vi "TORC Auto Shift.vi"(6 "RightMotorInput":dbl, 8 "Left Motor Input":dbl format="%#_13g", 9 "Velocity":dbl format="%#_13g", 10 "Throttle":dbl format="%#_13g", 11 "Time Met":bool) -> (3 "Shift Indicator":T1)   [LabVIEW 2015]
uses:
  Shift Enum.ctl
  Team Code/Robot Global Data.vi
  <vilib>/Rock Robotics/WPI/DriverStation/WPI_DriverStationRobotMode2.ctl
panel:
  out "Acceleration Chart":dbl(graph)
  in  "Coast_Speed_Limit":dbl=1.0
  in  "Coast_Throttle_Limit":dbl=0.1
  in  "Dropkik_Speed_Limit":dbl=3.0
  in  "Dropkik_Throttle_limit":dbl=0.3
  in  "Velocity_Upshift_Limit":dbl=3.25
  in  "Accel_up_limit":dbl
  in  "upshift_Thrtl_Limit":dbl=0.5
  in  "ShiftInterval":i32=500
  # "Original Upshift:\n3.75, changed to 3.25"
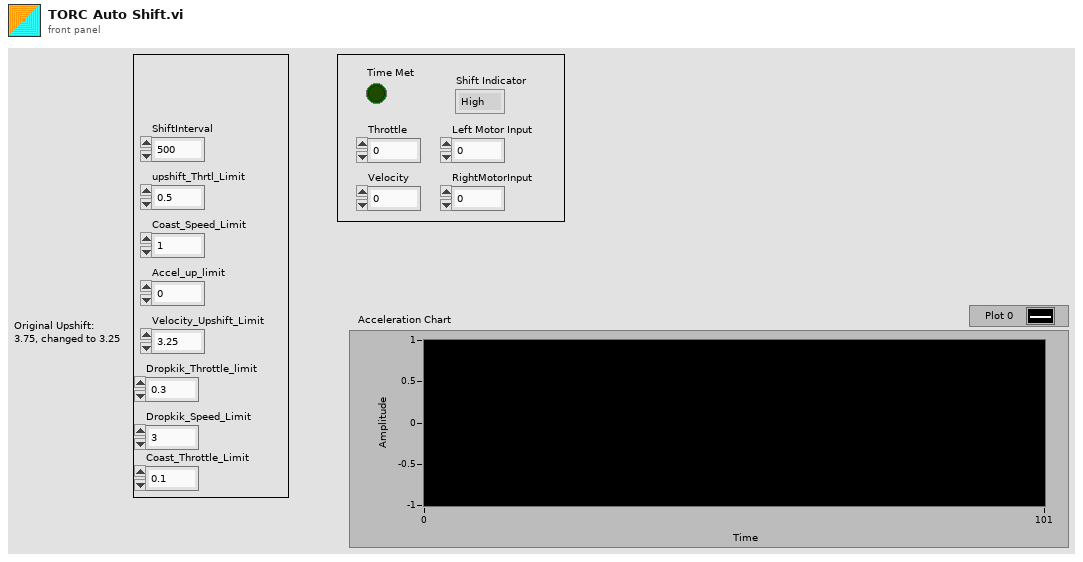
[diagram p1: front panel]
types:
  T1 = typedef "Shift Enum.ctl" = enum16{"High", "Low"}
  T2 = typedef "WPI_DriverStationRobotMode2.ctl" = enum16{"Autonomous Disabled", "Autonomous Enabled", "Teleop Disabled", "Teleop Enabled", "Disconnected", "Finish", "Test Disabled", "Test Enabled", "Emergency Stopped"}
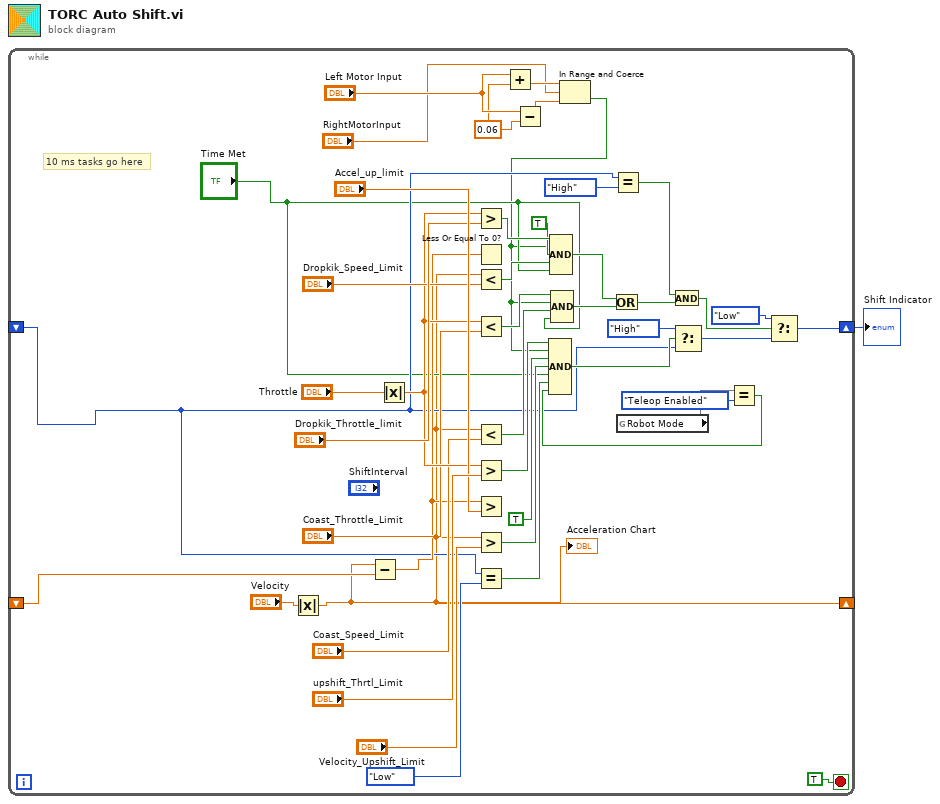
[diagram p0: block diagram]
diagram:
  n1 = while {
    shift-right: [w18] -> w1
    shift-left: _ -> [w11]
    shift-right: [w2] -> _
    shift-left: _ -> [w43]
    stop <- TRUE stop-if-true
    w6 = 0.06 ("y")
    # "10 ms tasks go here"
    n2 = Absolute Value(x="Velocity") -> (abs(x)=w2:dbl)
    "Acceleration Chart" <- w2
    n3 = Subtract(x=w2, y=w43) -> (x-y=w17:dbl)
    n4 = Absolute Value(x="Throttle") -> (abs(x)=w30:dbl)
    n5 = Greater?(x=w30, y="Dropkik_Throttle_limit") -> (0:w35:bool)
    n6 = Less Or Equal To 0?(x=w17) -> ()  [unwired: 1 out]
    n7 = Less?(x=w2, y="Dropkik_Speed_Limit") -> (x < y?=w32:bool)
    n8 = Less?(x=w30, y="Coast_Throttle_Limit") -> (x < y?=w31:bool)
    n9 = Less?(x=w2, y="Coast_Speed_Limit") -> (x < y?=w28:bool)
    n10 = Greater?(x=w30, y="upshift_Thrtl_Limit") -> (0:w44:bool)
    n11 = Greater?(x=w17, y="Accel_up_limit") -> ()  [unwired: 1 out]
    n12 = Greater?(x=w2, y="Velocity_Upshift_Limit") -> (0:w40:bool)
    n13 = Equal?(x=w11, y=Shift_Enum."Low") -> (x = y?=w38:bool)
    n14 = Add(x="Left Motor Input", y=w6) -> (x+y=w7:dbl)
    n15 = Subtract(x="Left Motor Input", y=w6) -> (x-y=w8:dbl)
    n16 = In Range and Coerce(upper limit=w7, x="RightMotorInput", lower limit=w8) -> (In Range?=w4:bool)  [unwired: 1 out]
    n17 = Compound Arithmetic op=AND(w35, w4, TRUE ("value"), w32, "Time Met") -> (w26:bool)
    n18 = Compound Arithmetic op=AND(w31, w4, w28, "Time Met") -> (w25:bool)
    n19 = Or(x=w26, y=w25) -> (x .or. y?=w24:bool)
    n20 = Equal?(x=w11, y=Shift_Enum."High") -> (x = y?=w23:bool)
    n21 = global read "Robot Global Data.vi" "Robot Mode"() -> (w14)
    n22 = And(x=w23, y=w24) -> (x .and. y?=w21:bool)
    n23 = Equal?(x=w14, y=WPI_DriverStationRobotMode2."Teleop Enabled") -> (x = y?=w12:bool)
    n24 = Compound Arithmetic op=AND(w44, w4, TRUE ("value"), w40, "Time Met", w38, w12) -> (w37:bool)
    n25 = Select(t=Shift_Enum."High", s=w37, f=w11) -> (s? t:f=w20:T1)
    n26 = Select(t=Shift_Enum."Low", s=w21, f=w20) -> (s? t:f=w18:T1)
  }
  "Shift Indicator" <- w1
